vi "AWG_commands.vi"(1 "Value":dbl, 2 "Channel":i32, 3 "Commands":T1(ring)) -> (0 "Comannd string":string)   [LabVIEW 2013]
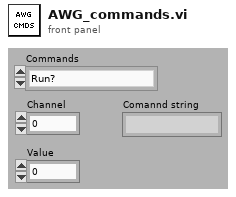
[diagram p1: front panel]
types:
  T1 = enum16{"Run?", "All output on?", "Run mode", "Sampling frequency", "Trigger", "Event", "Ch output on?", "Ch amplitude (V)", "Ch offset voltage (V)", "Ch marker1 high", "Ch marker1 low", "Ch marker1 delay", "Ch marker2 high", "Ch marker2 low", "Ch maker2 delay", "Ch skew"}
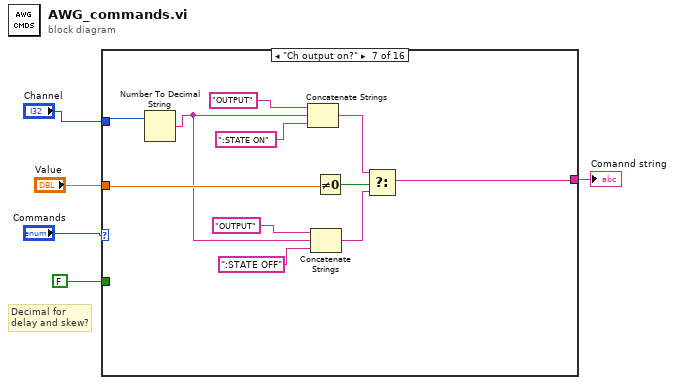
[diagram p0: block diagram]
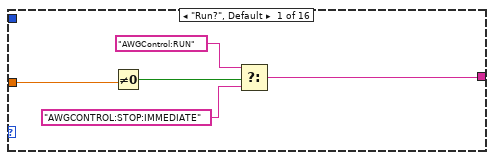
[diagram p2: hidden frame]
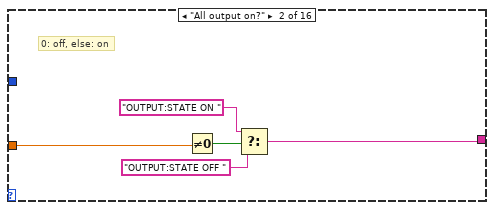
[diagram p3: hidden frame]
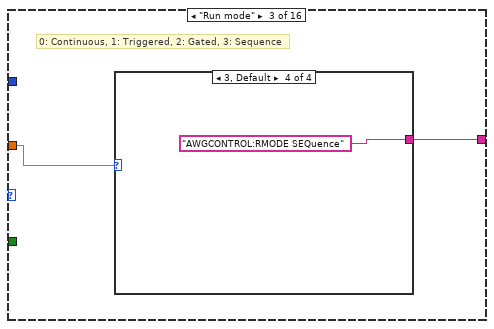
[diagram p4: hidden frame]
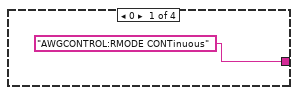
[diagram p5: hidden frame]
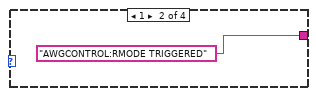
[diagram p6: hidden frame]
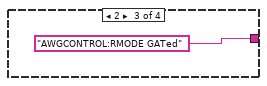
[diagram p7: hidden frame]
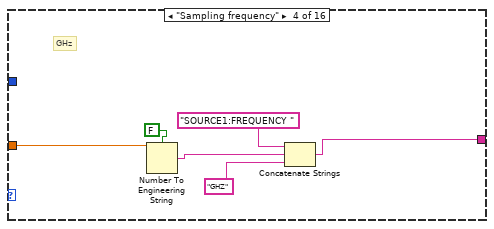
[diagram p8: hidden frame]
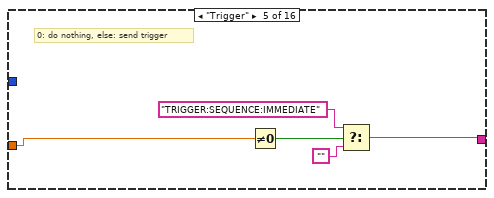
[diagram p9: hidden frame]
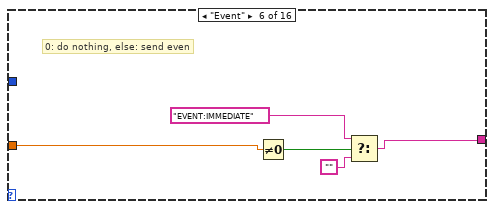
[diagram p10: hidden frame]
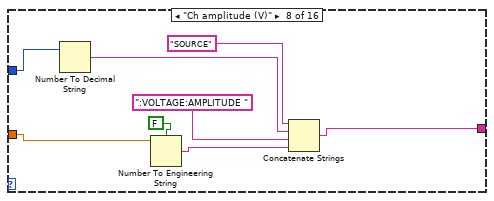
[diagram p11: hidden frame]
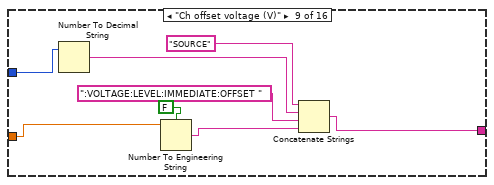
[diagram p12: hidden frame]
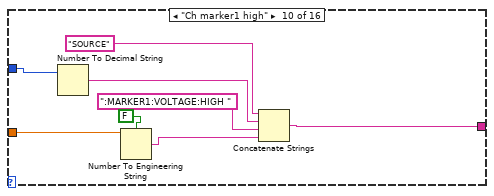
[diagram p13: hidden frame]
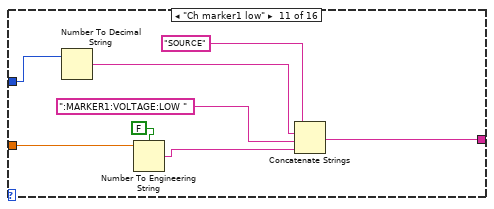
[diagram p14: hidden frame]
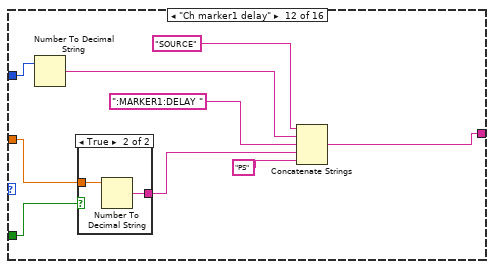
[diagram p15: hidden frame]
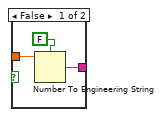
[diagram p16: hidden frame]
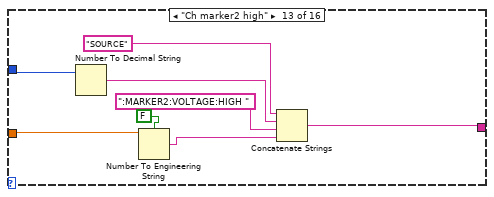
[diagram p17: hidden frame]
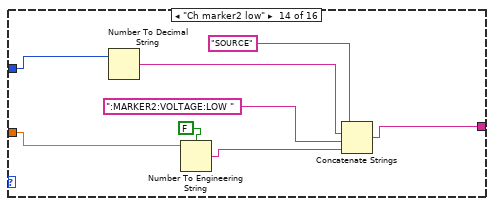
[diagram p18: hidden frame]
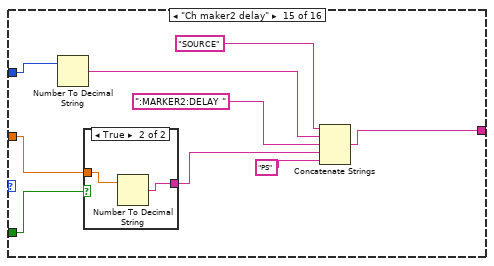
[diagram p19: hidden frame]
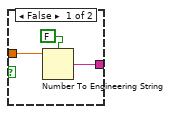
[diagram p20: hidden frame]
diagram:
  # "Decimal for\ndelay and skew?"
  n1 = case shown="\"Ch output on?\"" "Commands" {
    tunnel: "Value" -> [w10 w13 w17 w23 w30 w35 w47 w53 w60 w69 w77 w87 w97 w104 w114 w127]
    tunnel: [w6 w12 w16 w22 w29 w33 w46 w52 w61 w68 w78 w86 w95 w105 w112 w126] -> w3
    tunnel: "Channel" -> [_ _ _ _ _ _ w42 w50 w57 w67 w75 w84 w96 w103 w113 w130]
    tunnel: FALSE -> [_ _ _ _ _ _ _ _ _ _ _ w81 _ _ w111 w125]
    frame "Run?", Default {
      n2 = Not Equal To 0?(x=w10) -> (x != 0?=w9:bool)
      n3 = Select(t="AWGControl:RUN", s=w9, f="AWGCONTROL:STOP:IMMEDIATE") -> (s? t:f=w6:string)
    }
    frame "All output on?" {
      # "0: off, else: on"
      n4 = Not Equal To 0?(x=w13) -> (x != 0?=w14:bool)
      n5 = Select(t="OUTPUT:STATE ON ", s=w14, f="OUTPUT:STATE OFF ") -> (s? t:f=w12:string)
    }
    frame "Run mode" {
      # "0: Continuous, 1: Triggered, 2: Gated, 3: Sequence"
      n6 = case shown="3, Default" w17 {
        tunnel: ["AWGCONTROL:RMODE CONTinuous" "AWGCONTROL:RMODE TRIGGERED" "AWGCONTROL:RMODE GATed" "AWGCONTROL:RMODE SEQuence"] -> w16
        frame 0 {
        }
        frame 1 {
        }
        frame 2 {
        }
        frame 3, Default {
        }
      }
    }
    frame "Sampling frequency" {
      # "GHz"
      n7 = Number To Engineering String(1:FALSE, 4:w23) -> (0:w24:string)  [unwired: 2 in]
      n8 = Concatenate Strings("SOURCE1:FREQUENCY ", w24, "GHZ") -> (w22:string)
    }
    frame "Trigger" {
      # "0: do nothing, else: send trigger"
      n9 = Not Equal To 0?(x=w30) -> (x != 0?=w31:bool)
      n10 = Select(t="TRIGGER:SEQUENCE:IMMEDIATE", s=w31, f="") -> (s? t:f=w29:string)
    }
    frame "Event" {
      # "0: do nothing, else: send even"
      n11 = Not Equal To 0?(x=w35) -> (x != 0?=w37:bool)
      n12 = Select(t="EVENT:IMMEDIATE", s=w37, f="") -> (s? t:f=w33:string)
    }
    frame "Ch output on?" {
      n13 = Number To Decimal String(number=w42) -> (decimal integer string=w39:string)  [unwired: 1 in]
      n14 = Concatenate Strings("OUTPUT", w39, ":STATE ON") -> (w43:string)
      n15 = Concatenate Strings("OUTPUT", w39, ":STATE OFF") -> (w38:string)
      n16 = Not Equal To 0?(x=w47) -> (x != 0?=w48:bool)
      n17 = Select(t=w43, s=w48, f=w38) -> (s? t:f=w46:string)
    }
    frame "Ch amplitude (V)" {
      n18 = Number To Decimal String(number=w50) -> (decimal integer string=w49:string)  [unwired: 1 in]
      n19 = Number To Engineering String(1:FALSE, 4:w53) -> (0:w54:string)  [unwired: 2 in]
      n20 = Concatenate Strings("SOURCE", w49, ":VOLTAGE:AMPLITUDE ", w54) -> (w52:string)
    }
    frame "Ch offset voltage (V)" {
      n21 = Number To Decimal String(number=w57) -> (decimal integer string=w58:string)  [unwired: 1 in]
      n22 = Number To Engineering String(1:FALSE, 4:w60) -> (0:w62:string)  [unwired: 2 in]
      n23 = Concatenate Strings("SOURCE", w58, ":VOLTAGE:LEVEL:IMMEDIATE:OFFSET ", w62) -> (w61:string)
    }
    frame "Ch marker1 high" {
      n24 = Number To Decimal String(number=w67) -> (decimal integer string=w65:string)  [unwired: 1 in]
      n25 = Number To Engineering String(1:FALSE, 4:w69) -> (0:w70:string)  [unwired: 2 in]
      n26 = Concatenate Strings("SOURCE", w65, ":MARKER1:VOLTAGE:HIGH ", w70) -> (w68:string)
    }
    frame "Ch marker1 low" {
      n27 = Number To Decimal String(number=w75) -> (decimal integer string=w74:string)  [unwired: 1 in]
      n28 = Number To Engineering String(1:FALSE, 4:w77) -> (0:w79:string)  [unwired: 2 in]
      n29 = Concatenate Strings("SOURCE", w74, ":MARKER1:VOLTAGE:LOW ", w79) -> (w78:string)
    }
    frame "Ch marker1 delay" {
      n30 = Number To Decimal String(number=w84) -> (decimal integer string=w82:string)  [unwired: 1 in]
      n31 = case shown="True" w81 {
        tunnel: [w91 w93] -> w88
        tunnel: w87 -> [w90 w94]
        frame False {
          n32 = Number To Engineering String(1:FALSE, 4:w90) -> (0:w91:string)  [unwired: 2 in]
        }
        frame True {
          n33 = Number To Decimal String(number=w94) -> (decimal integer string=w93:string)  [unwired: 1 in]
        }
      }
      n34 = Concatenate Strings("SOURCE", w82, ":MARKER1:DELAY ", w88, "PS") -> (w86:string)
    }
    frame "Ch marker2 high" {
      n35 = Number To Decimal String(number=w96) -> (decimal integer string=w98:string)  [unwired: 1 in]
      n36 = Number To Engineering String(1:FALSE, 4:w97) -> (0:w100:string)  [unwired: 2 in]
      n37 = Concatenate Strings("SOURCE", w98, ":MARKER2:VOLTAGE:HIGH ", w100) -> (w95:string)
    }
    frame "Ch marker2 low" {
      n38 = Number To Decimal String(number=w103) -> (decimal integer string=w107:string)  [unwired: 1 in]
      n39 = Number To Engineering String(1:FALSE, 4:w104) -> (0:w109:string)  [unwired: 2 in]
      n40 = Concatenate Strings("SOURCE", w107, ":MARKER2:VOLTAGE:LOW ", w109) -> (w105:string)
    }
    frame "Ch maker2 delay" {
      n41 = Number To Decimal String(number=w113) -> (decimal integer string=w115:string)  [unwired: 1 in]
      n42 = case shown="True" w111 {
        tunnel: [w121 w124] -> w118
        tunnel: w114 -> [w120 w123]
        frame False {
          n43 = Number To Engineering String(1:FALSE, 4:w120) -> (0:w121:string)  [unwired: 2 in]
        }
        frame True {
          n44 = Number To Decimal String(number=w123) -> (decimal integer string=w124:string)  [unwired: 1 in]
        }
      }
      n45 = Concatenate Strings("SOURCE", w115, ":MARKER2:DELAY ", w118, "PS") -> (w112:string)
    }
    frame "Ch skew" {
      # "PS"
      n46 = case shown="True" w125 {
        tunnel: [w135 w137] -> w131
        tunnel: w127 -> [w134 w138]
        frame False {
          n47 = Number To Engineering String(1:FALSE, 4:w134) -> (0:w135:string)  [unwired: 2 in]
        }
        frame True {
          n48 = Number To Decimal String(number=w138) -> (decimal integer string=w137:string)  [unwired: 1 in]
        }
      }
      n49 = Number To Decimal String(number=w130) -> (decimal integer string=w129:string)  [unwired: 1 in]
      n50 = Concatenate Strings("SOURCE", w129, ":SKEW ", w131, "PS") -> (w126:string)
    }
  }
  "Comannd string" <- w3
